vi "Calc_Q.vi"(11 "P":dbl) -> (3 "Q":dbl)   [LabVIEW 2018]
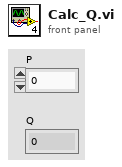
[diagram p1: front panel]
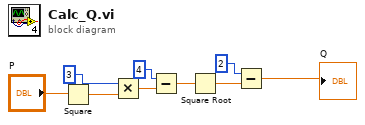
[diagram p0: block diagram]
diagram:
  n1 = Square(x="P") -> (x^2=w5:dbl)
  n2 = Multiply(x=3, y=w5) -> (x*y=w8:dbl)
  n3 = Subtract(x=4, y=w8) -> (x-y=w4:dbl)
  n4 = Square Root(x=w4) -> (sqrt(x)=w3:dbl)
  n5 = Subtract(x=2, y=w3) -> (x-y=→"Q":dbl)
